vi "Sequence-Stop tracking.vi"() -> (3 "MovCor Cluster ref out":refnum<vi>)   [LabVIEW 2020]
uses:
  Global Variables/gl_UI Ctrl Refs.vi
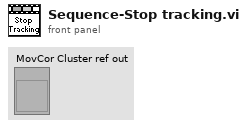
[diagram p1: front panel]
types:
  T1 = typedef "UI ctrl refs cluster.ctl" = cluster{"Top level VI path":path, "Top level VI ref":refnum<vi>, "User menu ref":refnum<k9>, "Sub Panel control":refnum<vi>, "Imaging Param Tab":refnum<vi>, "Occurrence-Start drivers":refnum<k4>, "Occurrence-Speed logging initialised":refnum<k4>, "Occurrence-XYZ stage initialised":refnum<k4>, "Exit button":refnum<vi>, "Status ind":refnum<vi>, "Set as origin":refnum<vi>, "Speed Logging":refnum<vi>, "Time Lapse":refnum<vi>, "Live Imaging":refnum<vi>, "AOL Z Stack":refnum<vi>, "Motor Z Stack":refnum<vi>, "Funct Acq button":refnum<vi>, "Hard Shutter":refnum<vi>, "Virtual Shutter":refnum<vi>, "Laser Power":refnum<vi>, "AOL Mode":refnum<vi>, "Frame Size":refnum<vi>, "Field of View":refnum<vi>, "Dwell Time":refnum<vi>, "Zoom":refnum<vi>, "AOL Z":refnum<vi>, "Objective":refnum<vi>, "Axis":refnum<vi>, "Paths & Names":refnum<vi>, "Experiment folder path (ind.)":refnum<vi>, "Last State (Ind.)":refnum<vi>, "Averages":refnum<vi>, "Angle (degrees)":refnum<vi>, "X centre":refnum<vi>, "Y centre":refnum<vi>, "Plane Mode":refnum<vi>, "# Planes":refnum<vi>, "Z Start":refnum<vi>, "Z Stop":refnum<vi>, "Z Step":refnum<vi>, "PMT 1":refnum<vi>, "PMT 2":refnum<vi>, "Stage XYZ Position":refnum<vi>, "Pockels@Z Start":refnum<vi>, "Pockels@Z Stop":refnum<vi>, "Obtain Z Start":refnum<vi>, "Obtain Z Stop":refnum<vi>, "Live stim.trig.period":refnum<vi>, "Live stim.trig.enable":refnum<vi>, "Movement Correction":refnum<vi>, "Load Reference Image":refnum<vi>, "XY Stage Move":refnum<vi>, "MovCor Cluster":refnum<vi>, "RefDAQParam":refnum<vi>, "Funct. Acq. Pockels Modulation":refnum<vi>, "Ref Laser Power":refnum<vi>, "Enable Video Recording":refnum<vi>, "Video Record-Live Imaging":refnum<vi>, "Video Record-Funct acq":refnum<vi>, "Reference Source":refnum<vi>, "AOL Z-stack Chirps Ready (ind)":refnum<vi>, "Target time between mov.cor. ref triggers (ms)":refnum<vi>, "Funct. Acq. Ref frame save":refnum<vi>, "Tracking button":refnum<vi>, "Show ref plots window":refnum<vi>, "Center freq ind (nm)":refnum<vi>, "Pickup mode (ind)":refnum<vi>, "Logging queue (ind)":refnum<vi>, "Back aperture power (ind.)":refnum<vi>, "Power after objective (ind.)":refnum<vi>, "Switch user":refnum<vi>, "Ls1 Conn. Status":refnum<vi>, "Ls1Tuning Status":refnum<vi>, "Ls1 Faults":refnum<vi>, "Ls1 Connection":refnum<vi>, "Ls1 Mode":refnum<vi>, "Ls1 POWER [mW]":refnum<vi>, "Ls1Shutter":refnum<vi>, "Ls1 Wavelength":refnum<vi>, "Ls1 Note":refnum<vi>, "Ls1 Confirm Wav":refnum<vi>, "Ls1 PreChrp Prism1":refnum<vi>, "Ls1 PreChrp Prism2":refnum<vi>, "Ls1 wav top Ind":refnum<vi>, "Ls1 power top Ind":refnum<vi>, "Ls1 Pump peak Hold":refnum<vi>, "Ls1 Status Ind":refnum<vi>, "Ls1 wav cancel":refnum<vi>, "Experiment Type":refnum<vi>, "Biology Information":refnum<vi>, "Camera recording status":refnum<vi>}
  T2 = typedef "test_fpga_control.ctl" = cluster{"x_offset_host":fxp<+/-,16,8>, "y_offset_host":fxp<+/-,16,8>, "use host offset":bool, "Set_Ref_Centroid":bool, "OldChirpCode":bool, "use array of offsets":bool, "x_offset_host array":fxp<+/-,16,8>[], "y_offset_host array ":fxp<+/-,16,8>[], "use host offset Z":bool, "swap Z":bool, "z_offset_host ":fxp<+/-,16,8>}
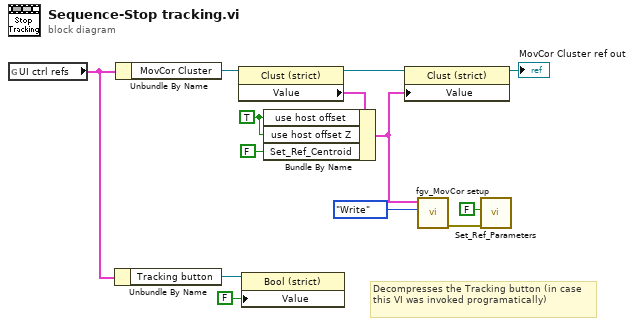
[diagram p0: block diagram]
diagram:
  w1 = TRUE ("use host offset")
  # "Decompresses the Tracking button (in case this VI was invoked programatically)"
  n1 = global read "gl_UI Ctrl Refs.vi" "UI ctrl refs"() -> (w3:T1)
  n2 = Unbundle By Name(w3) -> ("Tracking button"=w5:refnum<vi>)
  n3 = Unbundle By Name(w3) -> ("MovCor Cluster"=w8:refnum<vi>)
  n4 = property on="Property Node" class="Clust (strict)"(reference=w8) -> (reference out=w11:refnum<vi>, "Value"=w10:T2)  [unwired: 1 in, 1 out]
  n5 = property on="Property Node" class="Bool (strict)"(reference=w5, "Value"=FALSE) -> ()  [unwired: 1 in, 2 out]
  n6 = Bundle By Name(cluster=w10, "use host offset"=w1, "use host offset Z"=w1, "Set_Ref_Centroid"=FALSE) -> (w12:T2)
  n7 = property on="Property Node" class="Clust (strict)"(reference=w11, "Value"=w12) -> (reference out=→"MovCor Cluster ref out":refnum<vi>)  [unwired: 1 in, 1 out]
  n8 = call "fgv_MovCor setup.vi"("Status"=enum16{"Initialize", "Write", "Read"}."Write", "MovCor Cluster"=w12) -> ("error out"=w6:errorcluster)  [unwired: 8 in, 1 out]
  n9 = call "Set_Ref_Parameters.vi"("error in"=w6, "use_increment_halfrate"=FALSE) -> ()  [unwired: 7 in, 3 out]
